vi "Compile Datalog Array sub_VI.vi"(2 "XY Cluster":T1={"X Data"={"Complete?"=FALSE, "Motor Params"={"Duty %"=0.0, "X Freq"=0.0, "FWD/RVS"=FALSE}, "State"=enum."Stop", "Input"={"Coord Target"=0.0, "Tol"=0.0, "Accel"=0.0, "Decel"=0.0, "Max Speed"=0.0}, "Path"={"Speed plan"=[], "Profile"=enum."Triangular", "Max Speed"=0.0}, "PID"={"Kc"=0.0, "Ti"=0.0, "Td"=0.0}, "Motion"={"Speed"=0.0, "Dist"=0.0, "Accel"=0.0, "Dist Remain"=0.0}, "Time step i"=0}, "Y Data"={"Complete?"=FALSE, "Motor Params"={"Duty %"=0.0, "Freq"=0.0, "FWD/RVS"=FALSE}, "State"=enum."Stop", "Path"={"Speed plan"=[], " Profile"=enum."Triangular", "Max Speed"=0.0}, "PID"={"Kc"=0.0, "Ti"=0.0, "Td"=0.0}, "Motion"={"Speed"=0.0, "Dist"=0.0, "Accel"=0.0, "Dist Remain"=0.0}, "Input"={"Coord Target"=0.0, "Tol"=0.0, "Accel"=0.0, "Decel"=0.0, "Max Speed"=0.0}, "Time step i"=0}, "Timing"={"Runtime"=0.0, "Loop time"=0.0, "Loop iter"=0, "Tick"=0.0}, "stop"=FALSE} {"Y Data"."PID"."Ti" min=0.0; "X Data"."Input"."Tol" min=0.0}, 3 "Initialised Array":string[][](array[string])) -> (0 "Data Array":string[][](array[string]))   [LabVIEW 2017]
uses:
  XY Cluster.ctl
  Motor Status Enum.ctl
  Motion Type Def.ctl
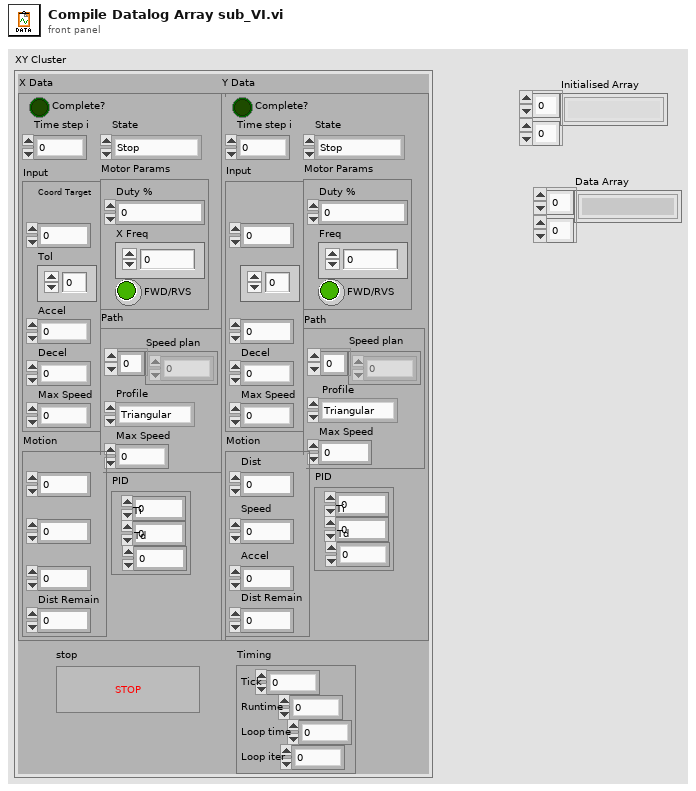
[diagram p1: front panel]
types:
  T1 = typedef "XY Cluster.ctl" = cluster{"X Data":cluster{"Complete?":bool, "Motor Params":cluster{"Duty %":dbl, "X Freq":dbl, "FWD/RVS":bool}, "State":T2, "Input":cluster{"Coord Target":dbl, "Tol":dbl, "Accel":dbl, "Decel":dbl, "Max Speed":dbl}, "Path":cluster{"Speed plan":dbl[], "Profile":T3, "Max Speed":dbl}, "PID":cluster{"Kc":dbl, "Ti":dbl, "Td":dbl}, "Motion":cluster{"Speed":dbl, "Dist":dbl, "Accel":dbl, "Dist Remain":dbl}, "Time step i":i32}, "Y Data":cluster{"Complete?":bool, "Motor Params":cluster{"Duty %":dbl, "Freq":dbl, "FWD/RVS":bool}, "State":T2, "Path":cluster{"Speed plan":dbl[], " Profile":T3, "Max Speed":dbl}, "PID":cluster{"Kc":dbl, "Ti":dbl, "Td":dbl}, "Motion":cluster{"Speed":dbl, "Dist":dbl, "Accel":dbl, "Dist Remain":dbl}, "Input":cluster{"Coord Target":dbl, "Tol":dbl, "Accel":dbl, "Decel":dbl, "Max Speed":dbl}, "Time step i":i32}, "Timing":cluster{"Runtime":dbl, "Loop time":dbl, "Loop iter":i32, "Tick":dbl}, "stop":bool}
  T2 = typedef "Motor Status Enum.ctl" = enum16{"Read PC", "Stop", "Move"}
  T3 = typedef "Motion Type Def.ctl" = enum16{"Trapezodial", "Triangular"}
  T4 = cluster{"Complete?":bool, "Motor Params":cluster{"Duty %":dbl, "X Freq":dbl, "FWD/RVS":bool}, "State":T2, "Input":cluster{"Coord Target":dbl, "Tol":dbl, "Accel":dbl, "Decel":dbl, "Max Speed":dbl}, "Path":cluster{"Speed plan":dbl[], "Profile":T3, "Max Speed":dbl}, "PID":cluster{"Kc":dbl, "Ti":dbl, "Td":dbl}, "Motion":cluster{"Speed":dbl, "Dist":dbl, "Accel":dbl, "Dist Remain":dbl}, "Time step i":i32}
  T5 = cluster{"Complete?":bool, "Motor Params":cluster{"Duty %":dbl, "Freq":dbl, "FWD/RVS":bool}, "State":T2, "Path":cluster{"Speed plan":dbl[], " Profile":T3, "Max Speed":dbl}, "PID":cluster{"Kc":dbl, "Ti":dbl, "Td":dbl}, "Motion":cluster{"Speed":dbl, "Dist":dbl, "Accel":dbl, "Dist Remain":dbl}, "Input":cluster{"Coord Target":dbl, "Tol":dbl, "Accel":dbl, "Decel":dbl, "Max Speed":dbl}, "Time step i":i32}
  T6 = cluster{"Runtime":dbl, "Loop time":dbl, "Loop iter":i32}
  T7 = cluster{i16, i16, "Duty %":dbl, "X Freq":dbl, "Numeric":dbl, "Speed":dbl, "Accel":dbl, "State":T2, "Coord Target":dbl, "Dist Remain":dbl, "Tol":dbl, "Profile":T3, "Max Speed":dbl, "Kc":dbl, "Ti":dbl, "Td":dbl}
  T8 = cluster{i16, i16, "Duty %":dbl, "Freq":dbl, "Numeric":dbl, "Speed":dbl, "Accel":dbl, "State":T2, "Coord Target":dbl, "Dist Remain":dbl, "Tol":dbl, " Profile":T3, "Max Speed":dbl, "Kc":dbl, "Ti":dbl, "Td":dbl}
  T9 = cluster{"Runtime":string, "Loop time":string, "Loop iter":string}
  T10 = cluster{string, string, "Duty %":string, "X Freq":string, "Numeric":string, "Speed":string, "Accel":string, string, "Coord Target":string, "Dist Remain":string, "Tol":string, string, "Max Speed":string, "Kc":string, "Ti":string, "Td":string}
  T11 = cluster{string, string, "Duty %":string, "Freq":string, "Numeric":string, "Speed":string, "Accel":string, string, "Coord Target":string, "Dist Remain":string, "Tol":string, string, "Max Speed":string, "Kc":string, "Ti":string, "Td":string}
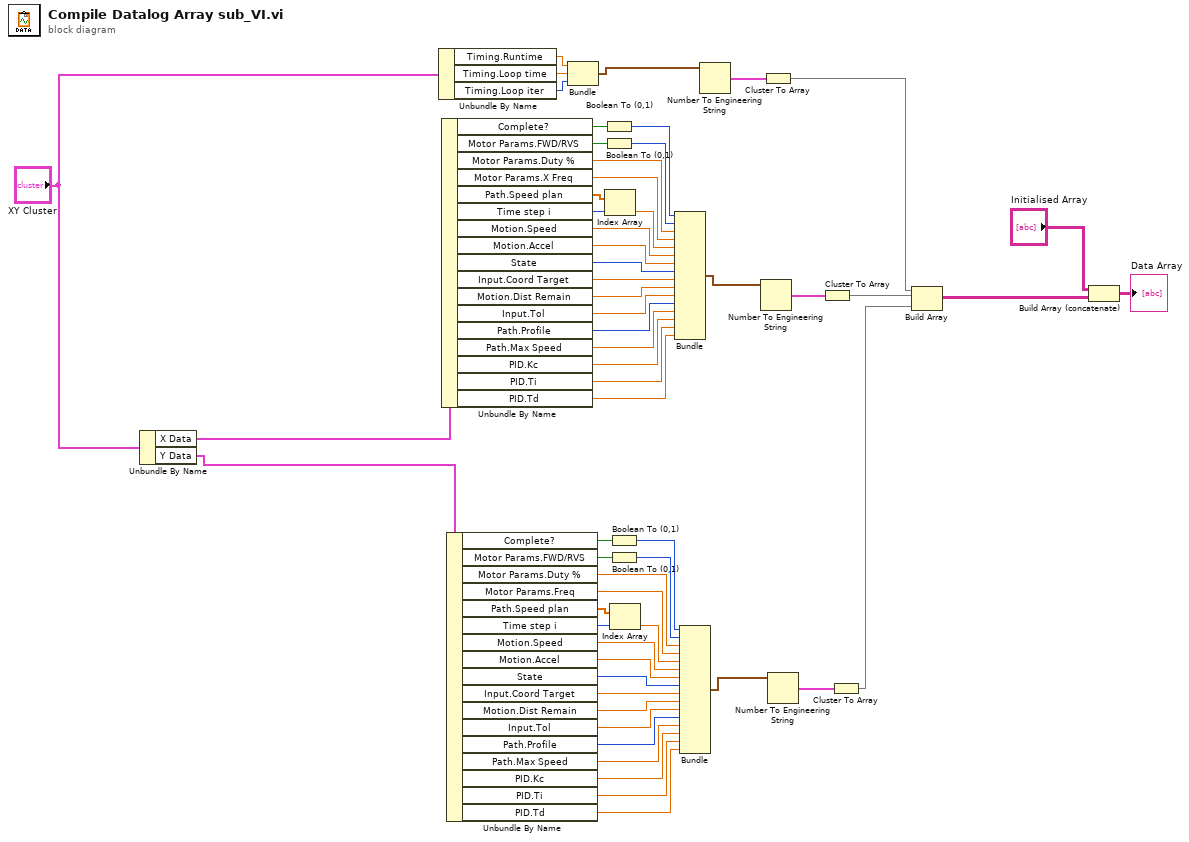
[diagram p0: block diagram]
diagram:
  n1 = Unbundle By Name("XY Cluster") -> ("X Data"=w52:T4, "Y Data"=w3:T5)
  n2 = Unbundle By Name("XY Cluster") -> ("Timing.Runtime"=w56:dbl, "Timing.Loop time"=w55:dbl, "Timing.Loop iter"=w54:i32)
  n3 = Unbundle By Name(w52) -> ("Complete?"=w51:bool, "Motor Params.FWD/RVS"=w50:bool, "Motor Params.Duty %"=w49:dbl, "Motor Params.X Freq"=w48:dbl, "Path.Speed plan"=w39:dbl[], "Time step i"=w38:i32, "Motion.Speed"=w36:dbl, "Motion.Accel"=w35:dbl, "State"=w34:T2, "Input.Coord Target"=w33:dbl, "Motion.Dist Remain"=w32:dbl, "Input.Tol"=w31:dbl, "Path.Profile"=w30:T3, "Path.Max Speed"=w29:dbl, "PID.Kc"=w28:dbl, "PID.Ti"=w27:dbl, "PID.Td"=w26:dbl)
  n4 = Unbundle By Name(w3) -> ("Complete?"=w23:bool, "Motor Params.FWD/RVS"=w22:bool, "Motor Params.Duty %"=w21:dbl, "Motor Params.Freq"=w20:dbl, "Path.Speed plan"=w17:dbl[], "Time step i"=w16:i32, "Motion.Speed"=w14:dbl, "Motion.Accel"=w13:dbl, "State"=w12:T2, "Input.Coord Target"=w11:dbl, "Motion.Dist Remain"=w10:dbl, "Input.Tol"=w9:dbl, "Path.Profile"=w8:T3, "Path.Max Speed"=w7:dbl, "PID.Kc"=w6:dbl, "PID.Ti"=w5:dbl, "PID.Td"=w4:dbl)
  n5 = Bundle("Runtime"=w56, "Loop time"=w55, "Loop iter"=w54) -> (w47:T6)  [unwired: 1 in]
  n6 = Boolean To (0,1)(Boolean=w51) -> (0, 1=w45:i16)
  n7 = Boolean To (0,1)(Boolean=w50) -> (0, 1=w44:i16)
  n8 = Index Array(array=w39, index=w38) -> (element=w37:dbl)
  n9 = Boolean To (0,1)(Boolean=w23) -> (0, 1=w19:i16)
  n10 = Boolean To (0,1)(Boolean=w22) -> (0, 1=w18:i16)
  n11 = Index Array(array=w17, index=w16) -> (element=w15:dbl)
  n12 = Bundle(w45, w44, "Duty %"=w49, "X Freq"=w48, "Numeric"=w37, "Speed"=w36, "Accel"=w35, "State"=w34, "Coord Target"=w33, "Dist Remain"=w32, "Tol"=w31, "Profile"=w30, "Max Speed"=w29, "Kc"=w28, "Ti"=w27, "Td"=w26) -> (w25:T7)  [unwired: 1 in]
  n13 = Bundle(w19, w18, "Duty %"=w21, "Freq"=w20, "Numeric"=w15, "Speed"=w14, "Accel"=w13, "State"=w12, "Coord Target"=w11, "Dist Remain"=w10, "Tol"=w9, "Profile"=w8, "Max Speed"=w7, "Kc"=w6, "Ti"=w5, "Td"=w4) -> (w2:T8)  [unwired: 1 in]
  n14 = Number To Engineering String(4:w47) -> (0:w46:T9)  [unwired: 3 in]
  n15 = Number To Engineering String(4:w25) -> (0:w24:T10)  [unwired: 3 in]
  n16 = Cluster To Array(cluster=w46) -> (array=w43:string[])
  n17 = Number To Engineering String(4:w2) -> (0:w42:T11)  [unwired: 3 in]
  n18 = Cluster To Array(cluster=w24) -> (array=w1:string[])
  n19 = Cluster To Array(cluster=w42) -> (array=w41:string[])
  n20 = Build Array(w43, w1, w41) -> (w40:string[][])
  n21 = Build Array (concatenate)("Initialised Array", w40) -> (→"Data Array":string[][])
